vi "señal discreta.vi"() -> ()   [LabVIEW 2016]
panel:
  in  "Array 3":dbl[](array[numeric])
  in  "x0 3":dbl
  in  "dx 3":dbl
  in  "Array 2":dbl[](array[numeric])
  in  "x0 2":dbl
  in  "dx 2":dbl
  in  "dx":dbl
  in  "x0":dbl
  out "Waveform Graph":T1(graph)
  in  "Array":dbl[](array[numeric])
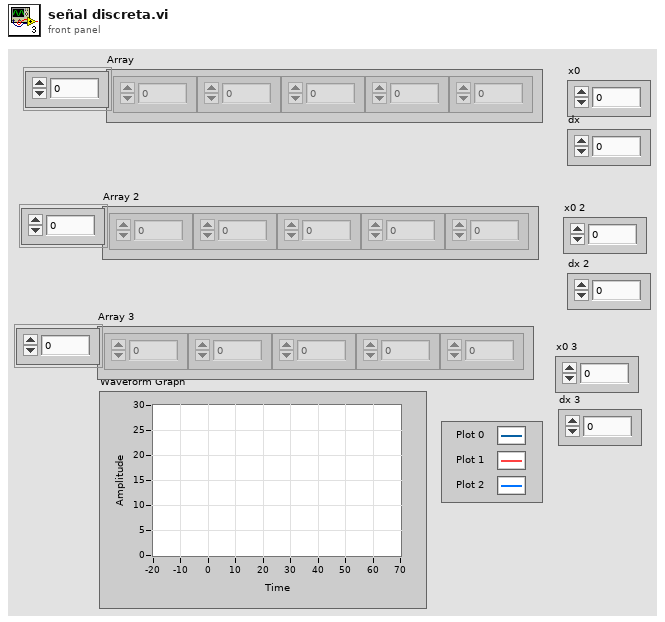
[diagram p1: front panel]
types:
  T1 = cluster{"x0 3":dbl, "dx 3":dbl, "Array 3":dbl[]}[]
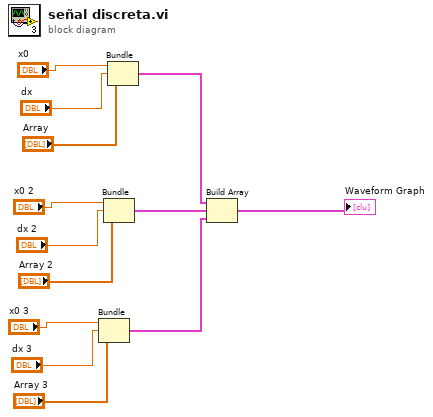
[diagram p0: block diagram]
diagram:
  n1 = Bundle("x0 3"="x0 3", "dx 3"="dx 3", "Array 3"="Array 3") -> (w2:cluster{"x0 3":dbl, "dx 3":dbl, "Array 3":dbl[]})  [unwired: 1 in]
  n2 = Bundle("x0 2"="x0 2", "dx 2"="dx 2", "Array 2"="Array 2") -> (w3:cluster{"x0 2":dbl, "dx 2":dbl, "Array 2":dbl[]})  [unwired: 1 in]
  n3 = Bundle("x0"="x0", "dx"="dx", "Array"="Array") -> (w4:cluster{"x0":dbl, "dx":dbl, "Array":dbl[]})  [unwired: 1 in]
  n4 = Build Array(w4, w3, w2) -> (→"Waveform Graph":T1)
